vi "dist.vi"(10 "y":dbl, 11 "x":dbl) -> (2 "d":dbl)   [LabVIEW 2009, in "LV_SLAM.lvlib"]
uses:
  LV_SLAM.lvlib
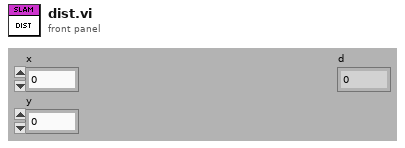
[diagram p1: front panel]
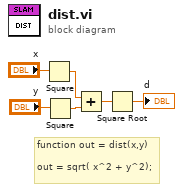
[diagram p0: block diagram]
diagram:
  # "function out = dist(x,y)\n\nout = sqrt( x^2 + y^2);"
  n1 = Square(x="x") -> (x^2=w5:dbl)
  n2 = Square(x="y") -> (x^2=w4:dbl)
  n3 = Add(x=w5, y=w4) -> (x+y=w6:dbl)
  n4 = Square Root(x=w6) -> (sqrt(x)=→"d":dbl)
